vi "数据处理整合(子VI).vi"   [LabVIEW 2016]
types:
  T1 = cluster{"总磷":string[][], "总氮":string[][], "多参数":string[][], "氨氮":string[][], "CODMn":string[][], "PH":string[][], "CODCr":string[][]}
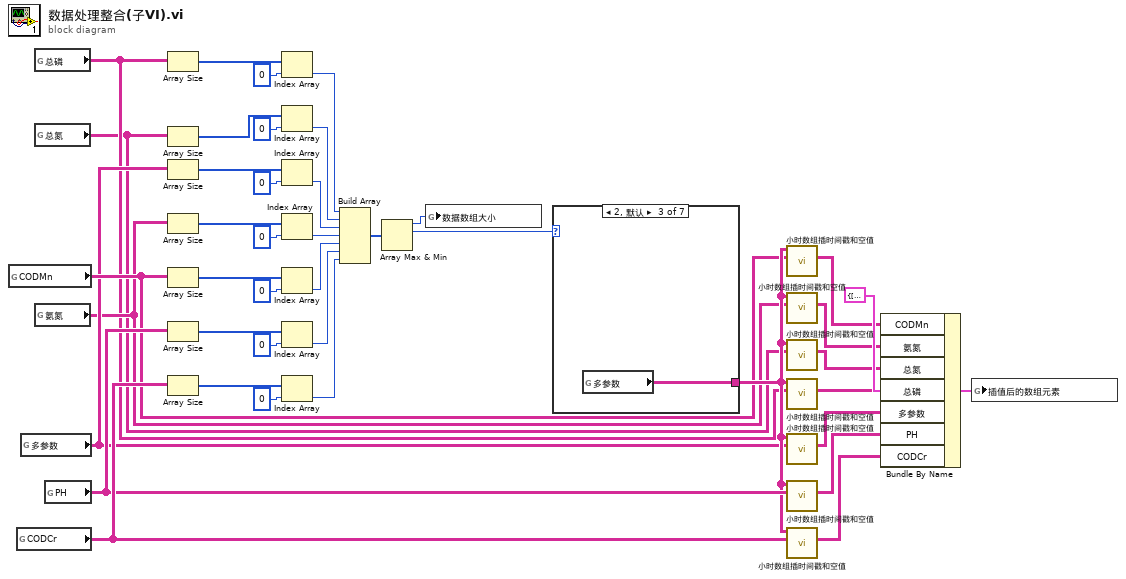
[diagram p0: block diagram]
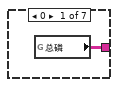
[diagram p2: hidden frame]
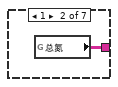
[diagram p3: hidden frame]
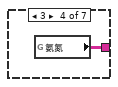
[diagram p4: hidden frame]
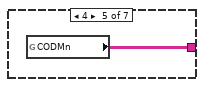
[diagram p5: hidden frame]
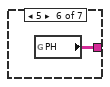
[diagram p6: hidden frame]
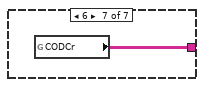
[diagram p7: hidden frame]
diagram:
  n1 = global read "全局 CODMn.vi" "CODMn"() -> (w27:string[][])
  n2 = global read "全局 所有参数.vi" "CODCr"() -> (w37:string[][])
  n3 = global read "全局 多参数.vi" "多参数"() -> (w26:string[][])
  n4 = global read "全局 总磷.vi" "总磷"() -> (w21:string[][])
  n5 = global read "全局 总氮.vi" "总氮"() -> (w19:string[][])
  n6 = global read "全局 氨氮.vi" "氨氮"() -> (w24:string[][])
  n7 = global read "全局 所有参数.vi" "PH"() -> (w36:string[][])
  n8 = Array Size(array=w21) -> (size(s)=w1:i32[])
  n9 = Array Size(array=w19) -> (size(s)=w4:i32[])
  n10 = Array Size(array=w26) -> (size(s)=w5:i32[])
  n11 = Array Size(array=w24) -> (size(s)=w8:i32[])
  n12 = Array Size(array=w27) -> (size(s)=w9:i32[])
  n13 = Array Size(array=w36) -> (size(s)=w39:i32[])
  n14 = Array Size(array=w37) -> (size(s)=w38:i32[])
  n15 = Index Array(array=w1, index=0 ("索引")) -> (element=w11:i32)
  n16 = Index Array(array=w4, index=0 ("索引")) -> (element=w12:i32)
  n17 = Index Array(array=w5, index=0 ("索引")) -> (element=w13:i32)
  n18 = Index Array(array=w8, index=0 ("索引")) -> (element=w14:i32)
  n19 = Index Array(array=w9, index=0 ("索引")) -> (element=w15:i32)
  n20 = Index Array(array=w39, index=0 ("索引")) -> (element=w40:i32)
  n21 = Index Array(array=w38, index=0 ("索引")) -> (element=w41:i32)
  n22 = Build Array(w11, w12, w13, w14, w15, w40, w41) -> (w16:i32[])
  n23 = Array Max & Min(array=w16) -> (max value=w17:i32, max index (indices)=w32:i32)  [unwired: 2 out]
  n24 = global write "全局 数据数组大小.vi" "数据数组大小"(w17) -> ()
  n25 = case shown="2, 默认" w32 {
    tunnel: [w42 w43 w44 w45 w46 w47 w48] -> w33
    frame 0 {
      n26 = global read "全局 总磷.vi" "总磷"() -> (w42:string[][])
    }
    frame 1 {
      n27 = global read "全局 总氮.vi" "总氮"() -> (w43:string[][])
    }
    frame 2, Default {
      n28 = global read "全局 多参数.vi" "多参数"() -> (w44:string[][])
    }
    frame 3 {
      n29 = global read "全局 氨氮.vi" "氨氮"() -> (w45:string[][])
    }
    frame 4 {
      n30 = global read "全局 CODMn.vi" "CODMn"() -> (w46:string[][])
    }
    frame 5 {
      n31 = global read "全局 所有参数.vi" "PH"() -> (w47:string[][])
    }
    frame 6 {
      n32 = global read "全局 所有参数.vi" "CODCr"() -> (w48:string[][])
    }
  }
  n33 = call "小时数组插时间戳和空值.vi"("多参数"=w33, "待插值"=w27) -> ("新输出"=w18:string[][])  [unwired: 8 in]
  n34 = call "小时数组插时间戳和空值.vi"("多参数"=w33, "待插值"=w24) -> ("新输出"=w25:string[][])  [unwired: 8 in]
  n35 = call "小时数组插时间戳和空值.vi"("多参数"=w33, "待插值"=w19) -> ("新输出"=w20:string[][])  [unwired: 8 in]
  n36 = call "小时数组插时间戳和空值.vi"("多参数"=w33, "待插值"=w21) -> ("新输出"=w22:string[][])  [unwired: 8 in]
  n37 = call "小时数组插时间戳和空值.vi"("多参数"=w33, "待插值"=w26) -> ("新输出"=w23:string[][])  [unwired: 8 in]
  n38 = call "小时数组插时间戳和空值.vi"("多参数"=w33, "待插值"=w36) -> ("新输出"=w35:string[][])  [unwired: 8 in]
  n39 = call "小时数组插时间戳和空值.vi"("多参数"=w33, "待插值"=w37) -> ("新输出"=w34:string[][])  [unwired: 8 in]
  n40 = Bundle By Name(cluster=T1 {"总磷"=[], "总氮"=[], "多参数"=[], "氨氮"=[], "CODMn"=[], "PH"=[], "CODCr"=[]} ("插值后的数组元素"), "CODMn"=w18, "氨氮"=w25, "总氮"=w20, "总磷"=w22, "多参数"=w23, "PH"=w35, "CODCr"=w34) -> (w29:T1)
  n41 = global write "插值后的新数组.vi" "插值后的数组元素"(w29) -> ()
